vi "draw object.vi"(9 "Object":T1, 11 "picture in":picture) -> (3 "picture out":picture)   [LabVIEW 2009]
uses:
  object.ctl
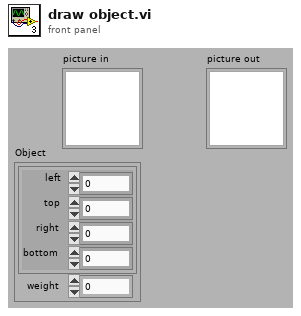
[diagram p1: front panel]
types:
  T1 = typedef "object.ctl" = cluster{"rect":cluster{"left":i16, "top":i16, "right":i16, "bottom":i16}, "weight":sgl}
  T2 = cluster{"left":i16, "top":i16, "right":i16, "bottom":i16}
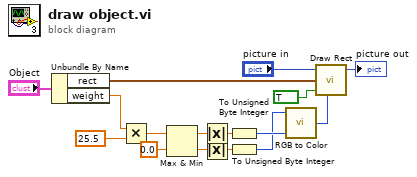
[diagram p0: block diagram]
diagram:
  n1 = Unbundle By Name("Object") -> ("rect"=w4:T2, "weight"=w3:sgl)
  n2 = Multiply(x=w3, y=25.5) -> (x*y=w15:dbl)
  n3 = Max & Min(x=w15, y=0.0) -> (max(x,y)=w13:dbl, min(x,y)=w12:dbl)
  n4 = Absolute Value(x=w13) -> (abs(x)=w11:dbl)
  n5 = Absolute Value(x=w12) -> (abs(x)=w10:dbl)
  n6 = To Unsigned Byte Integer(number=w11) -> (unsigned 8bit integer=w9:u8)
  n7 = To Unsigned Byte Integer(number=w10) -> (unsigned 8bit integer=w8:u8)
  n8 = call <vilib>:"RGB to Color.vi"("B"=w9, "R"=w8) -> ("Color"=w7:u32)  [unwired: 1 in]
  n9 = call <vilib>:"Draw Rect.vi"("picture"="picture in", "rect"=w4, "fill?(F)"=TRUE, "color(black)"=w7) -> ("new picture"=→"picture out":picture)  [unwired: 5 in]
